vi "Z Stack Code debug.vi"() -> ()   [LabVIEW 2020]
panel:
  in  "stop":bool
  out "Error out":errorcluster={"status"=TRUE, "code"=-2147218439, "source"="Exception occured in SPiiPlusCOM660.AsyncChannel.1: Code 3065, The command cannot be executed while the current motion is in progress in Z Stack Code debug.vi"}
  out "Connected":bool
  out "GetFirmwareVersion 2":string="3.03\r"
  in  "SPIIPLUSCOM660Lib.IAsyncChannel":refnum<k7>
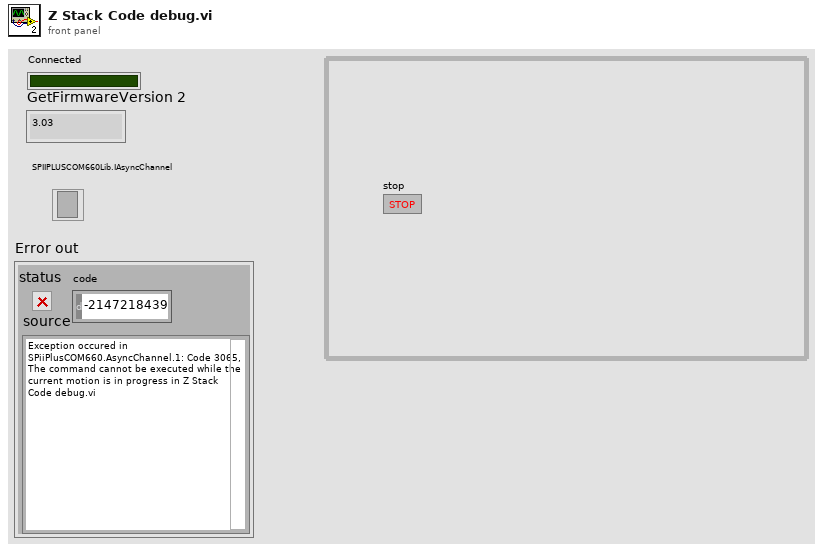
[diagram p1: front panel]
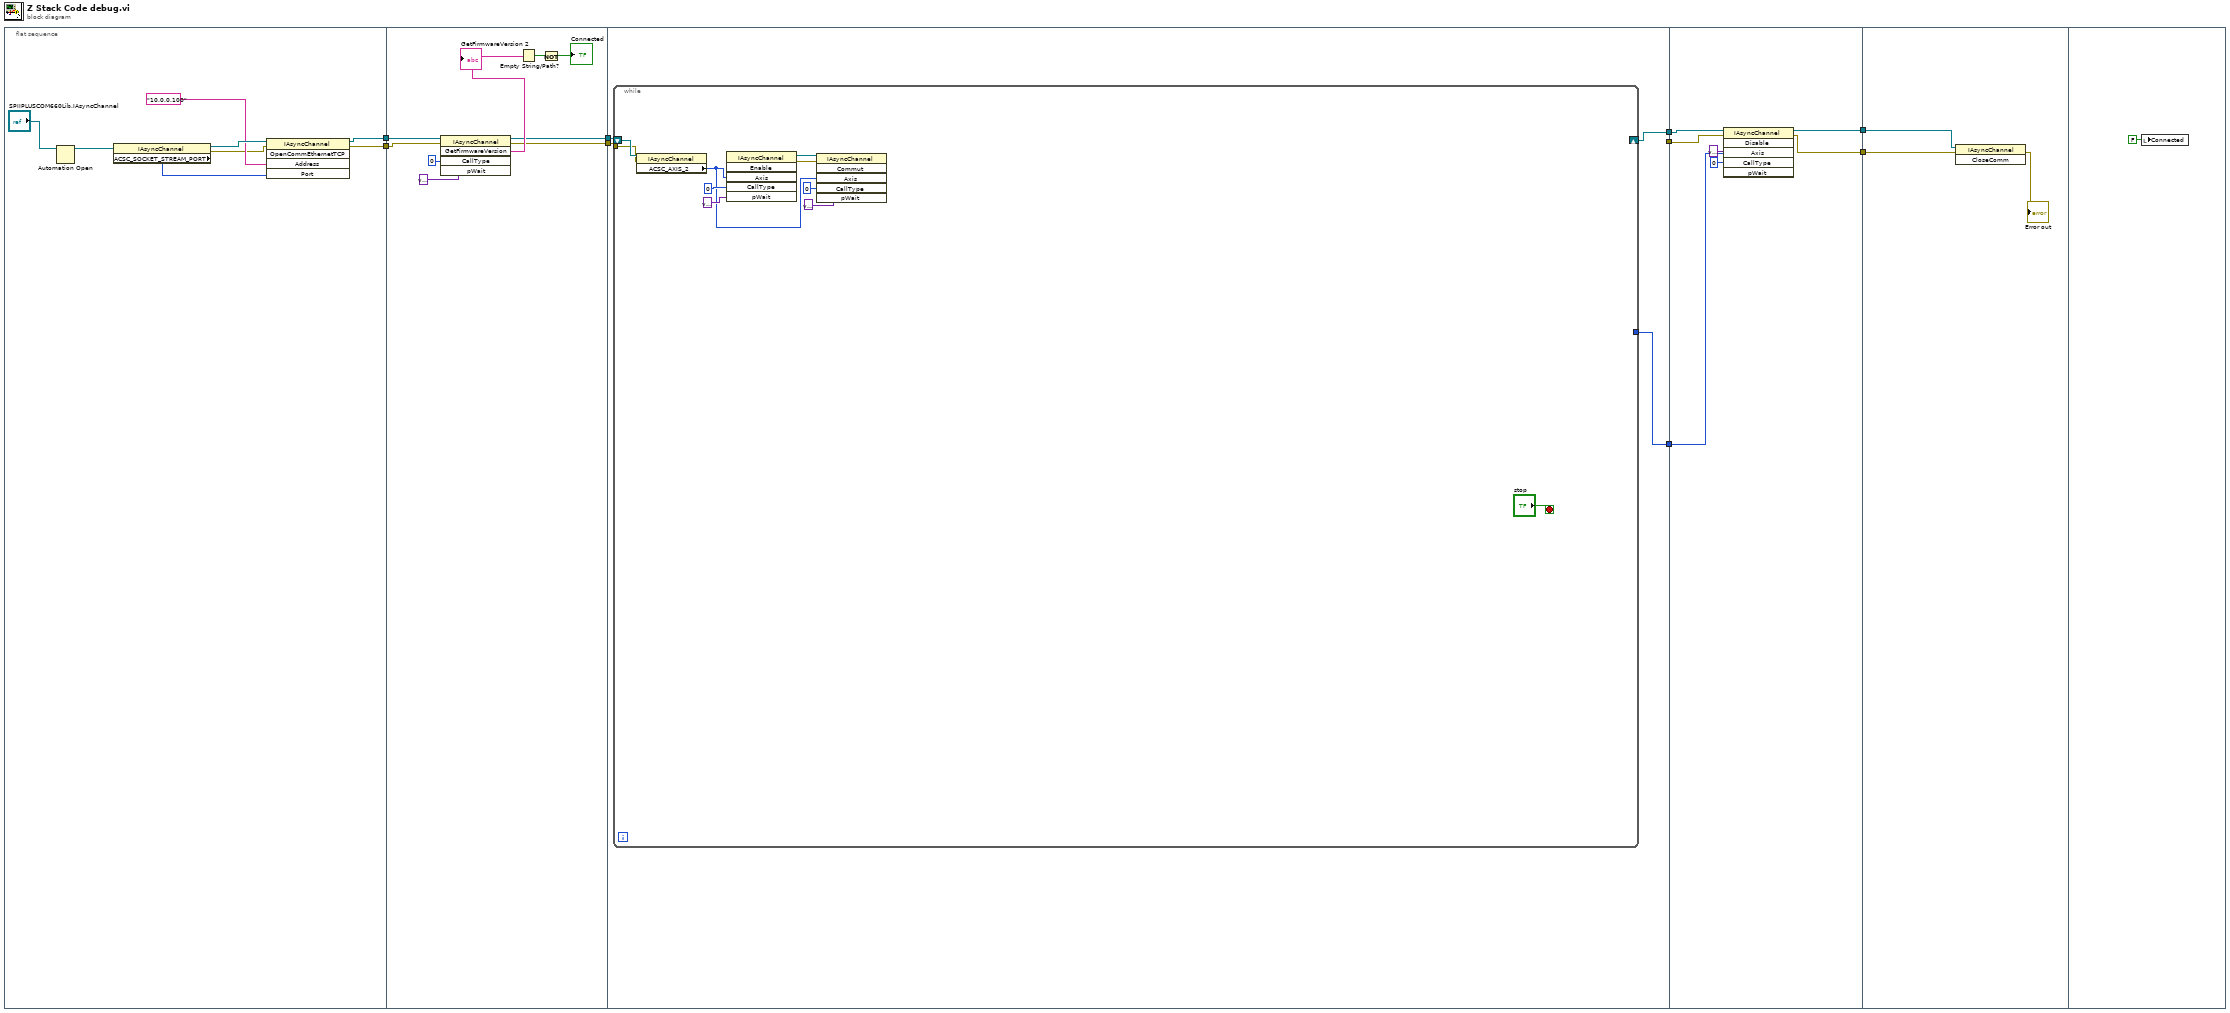
[diagram p0: block diagram]
diagram:
  n1 = flat-sequence {
    tunnel: [w12] -> w9
    tunnel: [w11] -> w8
    tunnel: w9 -> [w22]
    tunnel: w8 -> [w21]
    tunnel: [w19] -> w7
    tunnel: [w18] -> w6
    tunnel: w7 -> [w29]
    tunnel: w6 -> [w28]
    tunnel: [w27] -> w5
    tunnel: [_] -> w4
    tunnel: [w30] -> w1
    tunnel: w5 -> [w47]
    tunnel: w4 -> [w46]
    tunnel: [w45] -> w3
    tunnel: [w44] -> w2
    tunnel: w1 -> [w43]
    tunnel: w3 -> [w49]
    tunnel: w2 -> [w48]
    frame #0 {
      n2 = Automation Open(Automation Refnum="SPIIPLUSCOM660Lib.IAsyncChannel") -> (Automation Refnum=w17:refnum<k7>)  [unwired: 3 in, 1 out]
      n3 = property class="IAsyncChannel"(reference=w17) -> (reference out=w16:refnum<k7>, error out=w10:errorcluster, "ACSC_SOCKET_STREAM_PORT"=w14:i32)  [unwired: 1 in]
      n4 = invoke class="IAsyncChannel" method="OpenCommEthernetTCP"(reference=w16, error in=w10, "Address"="10.0.0.100", "Port"=w14) -> (reference out=w12:refnum<k7>, error out=w11:errorcluster)  [unwired: 1 in, 3 out]
    }
    frame #1 {
      n5 = invoke class="IAsyncChannel" method="GetFirmwareVersion"(reference=w22, error in=w21, "CallType"=u64 0, "pWait"=variant) -> (reference out=w19:refnum<k7>, error out=w18:errorcluster, "GetFirmwareVersion"=w24:string)  [unwired: 1 in, 2 out]
      "GetFirmwareVersion 2" <- w24
      n6 = Empty String/Path?(string/path=w24) -> (empty?=w23:bool)
      n7 = Not(x=w23) -> (.not. x?=→"Connected":bool)
    }
    frame #2 {
      n8 = while {
        tunnel: [_] -> w30
        tunnel: w28 -> [w34]
        shift-right: [_] -> w27
        shift-left: w29 -> [w35]
        stop <- "stop" stop-if-true
        n9 = property class="IAsyncChannel"(reference=w35, error in=w34) -> ("ACSC_AXIS_2"=w33:i32)  [unwired: 2 out]
        n10 = invoke class="IAsyncChannel" method="Enable"("Axis"=w33, "CallType"=u64 0, "pWait"=variant) -> (reference out=w37:refnum<k7>, error out=w36:errorcluster)  [unwired: 3 in, 4 out]
        n11 = invoke class="IAsyncChannel" method="Commut"(reference=w37, error in=w36, "Axis"=w33, "CallType"=u64 0, "pWait"=variant) -> ()  [unwired: 1 in, 6 out]
      }
    }
    frame #3 {
      n12 = invoke class="IAsyncChannel" method="Disable"(reference=w47, error in=w46, "Axis"=w43, "CallType"=u64 0, "pWait"=variant) -> (reference out=w45:refnum<k7>, error out=w44:errorcluster)  [unwired: 1 in, 4 out]
    }
    frame #4 {
      n13 = invoke class="IAsyncChannel" method="CloseComm"(reference=w49, error in=w48) -> (error out=→"Error out":errorcluster)  [unwired: 1 in, 2 out]
    }
    frame #5 {
      n14 = local write "Connected"(FALSE ("Connected")) -> ()
    }
  }
